vi "Dispatcher Error Offset.vi"() -> (3 "base error offset":i32)   [LabVIEW 2017]
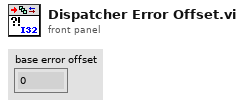
[diagram p1: front panel]
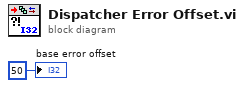
[diagram p0: block diagram]
diagram:
  "base error offset" <- 50 ("base error code")
